vi "Is Numeric.vi"(11 "input string":string) -> (3 "is numeric?":bool)   [LabVIEW 2020, in "UI Common.lvlib"]
uses:
  UI Common.lvlib
  <vilib>/regexp/Match Regular Expression.xnode
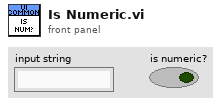
[diagram p1: front panel]
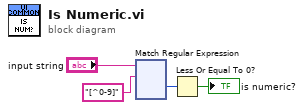
[diagram p0: block diagram]
diagram:
  n1 = xnode "Match Regular Expression"("input string"="input string", "regular expression"="[^0-9]") -> ("offset past match"=w1:i32)  [unwired: 4 in, 4 out]
  n2 = Less Or Equal To 0?(x=w1) -> (x <= 0?=→"is numeric?":bool)
